vi "Read_INI_File-Image_Proc.vi"(8 "ERROR IN":errorcluster, 11 "[IN] refnum - ini file":T1) -> (0 "ERROR OUT":errorcluster, 1 "[OUT] Minimal diameter":dbl, 3 "[OUT] Erosion Number":i32, 4 "[OUT] Maximal diameter":dbl, 5 "[OUT] Index for thresholding":i8)   [LabVIEW 2017]
doc: "This subVI reads two values in the *ini file - under the \"Image Processing Values\" section"
uses:
  <vilib>/Utility/config.llb/Config Data RefNum.ctl
  <vilib>/Utility/config.llb/Read Key (I32).vi
  <vilib>/Utility/config.llb/Read Key (Double).vi
  <vilib>/Utility/config.llb/NI_LVConfig.lvlib
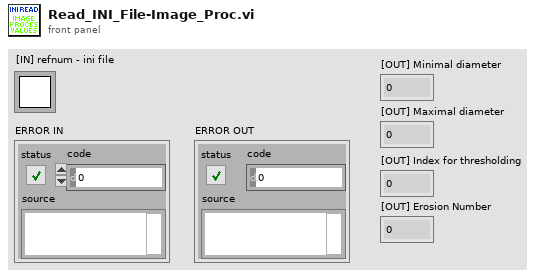
[diagram p1: front panel]
types:
  T1 = typedef "NI_LVConfig.lvlib/Config Data RefNum.ctl" = refnum<k1>
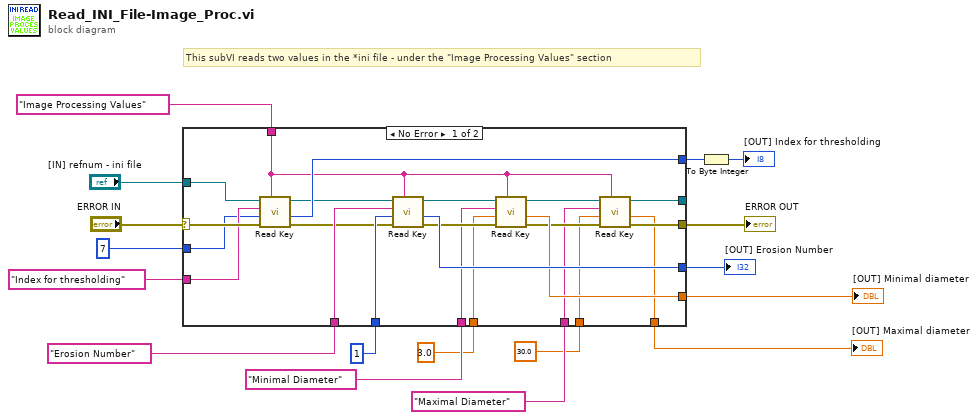
[diagram p0: block diagram]
diagram:
  # "This subVI reads two values in the *ini file - under the \"Image Processing Values\" section"
  n1 = case shown="No Error" "ERROR IN" {
    selector: "ERROR IN" -> [w40 w44]
    tunnel: "[IN] refnum - ini file" -> [w39 w45]
    tunnel: "Image Processing Values" ("section") -> [w22 _]
    tunnel: "Index for thresholding" ("key") -> [w38 _]
    tunnel: 7 ("default value") -> [w37 w46]
    tunnel: [w36 w46] -> w9
    tunnel: "Erosion Number" ("key") -> [w34 _]
    tunnel: 1 ("default value") -> [w33 w43]
    tunnel: [w21 w44] -> w10
    tunnel: [w23 w45] -> _
    tunnel: [w31 w43] -> w7
    tunnel: "Minimal Diameter" ("key") -> [w28 _]
    tunnel: 3.0 ("default value") -> [w27 w42]
    tunnel: [w26 w42] -> w4
    tunnel: "Maximal Diameter" ("key") -> [w20 _]
    tunnel: 30.0 ("default value") -> [w19 w41]
    tunnel: [w18 w41] -> w1
    frame No Error {
      n2 = call-poly <vilib>:"Read Key.vi"("section"=w22, "error in (no error)"=w40, "default value"=w37, "key"=w38, "refnum"=w39) -> ("error out"=w32:errorcluster, "value"=w36:i32, "refnum out"=w35:T1)  [unwired: 3 in, 1 out]
      n3 = call-poly <vilib>:"Read Key.vi"("section"=w22, "error in (no error)"=w32, "default value"=w33, "key"=w34, "refnum"=w35) -> ("error out"=w29:errorcluster, "value"=w31:i32, "refnum out"=w30:T1)  [unwired: 3 in, 1 out]
      n4 = call-poly <vilib>:"Read Key.vi"("section"=w22, "error in (no error)"=w29, "default value"=w27, "key"=w28, "refnum"=w30) -> ("error out"=w24:errorcluster, "value"=w26:dbl, "refnum out"=w25:T1)  [unwired: 3 in, 1 out]
      n5 = call-poly <vilib>:"Read Key.vi"("section"=w22, "error in (no error)"=w24, "default value"=w19, "key"=w20, "refnum"=w25) -> ("error out"=w21:errorcluster, "value"=w18:dbl, "refnum out"=w23:T1)  [unwired: 3 in, 1 out]
    }
    frame Error {
    }
  }
  "ERROR OUT" <- w10
  "[OUT] Erosion Number" <- w7
  "[OUT] Minimal diameter" <- w4
  "[OUT] Maximal diameter" <- w1
  n6 = To Byte Integer(number=w9) -> (8bit integer=→"[OUT] Index for thresholding":i8)
